vi "Main.vi"() -> ()   [LabVIEW 2022 SP3]
uses:
  <userlib>/_OpenG.lib/file/file.llb/Build Path - File Names Array__ogtk.vi
  <userlib>/_OpenG.lib/file/file.llb/Compare Two Paths - Scalar__ogtk.vi
  <userlib>/_OpenG.lib/file/file.llb/Build Path - Traditional - path__ogtk.vi
  <userlib>/_OpenG.lib/file/file.llb/Strip Path - Traditional__ogtk.vi
panel:
  in  "Status":string
  in  "Abort":bool
  out "Folder Stack":i32
  out "Current File":path
  out "Copied Count":i32
  out "Files Copied":path[](array[path])
  out "error out":errorcluster
  in  "Dest Folder":path=path "\\\\tyrian\\D/Literature/Comics/Marvel"
  in  "Local Folder":path=path "D:/Marvel"
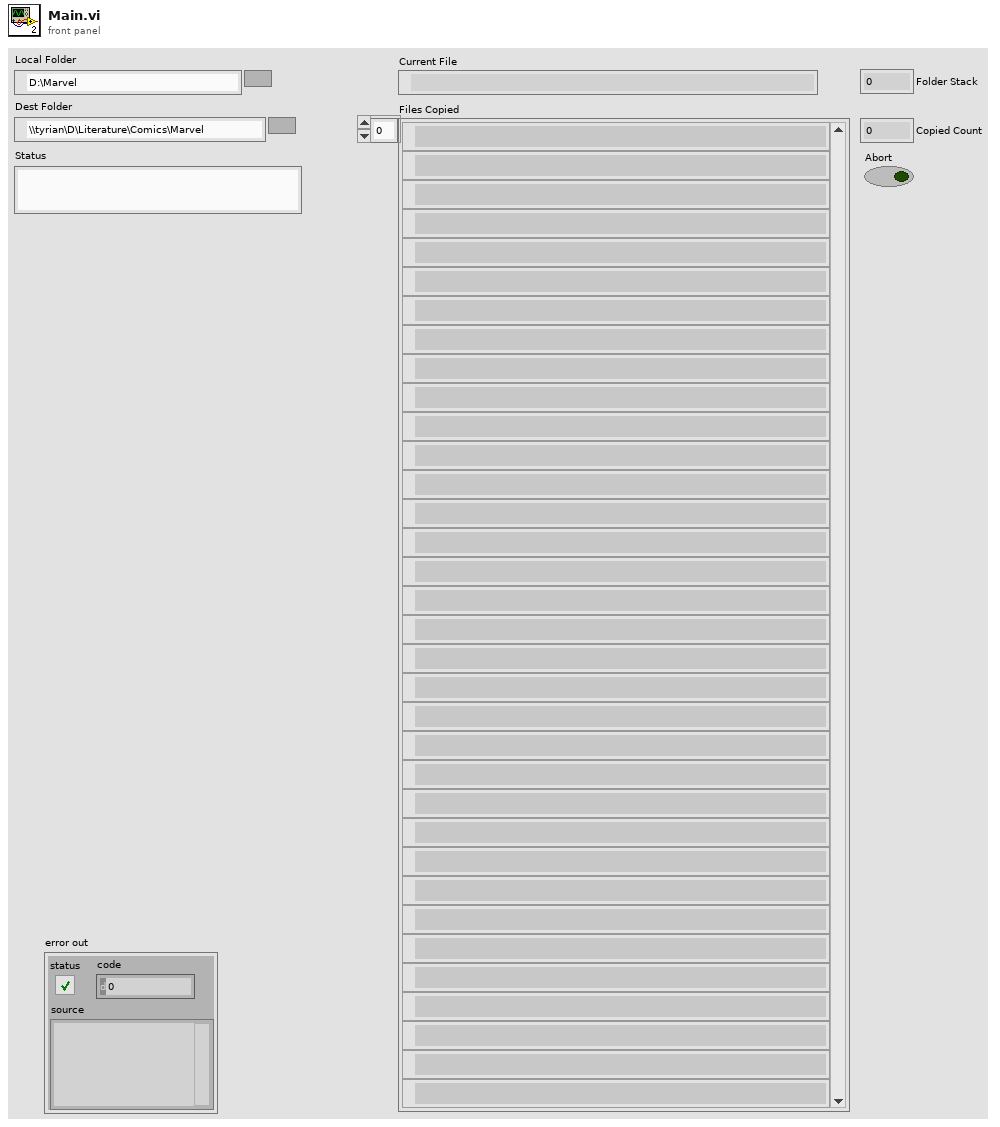
[diagram p1: front panel]
types:
  T1 = cluster{"Archive":bool, "Normal":bool, "Temporary":bool, "Compressed":bool, "Offline":bool, "Content Indexed":bool, "Encrypted (cannot set)":bool}
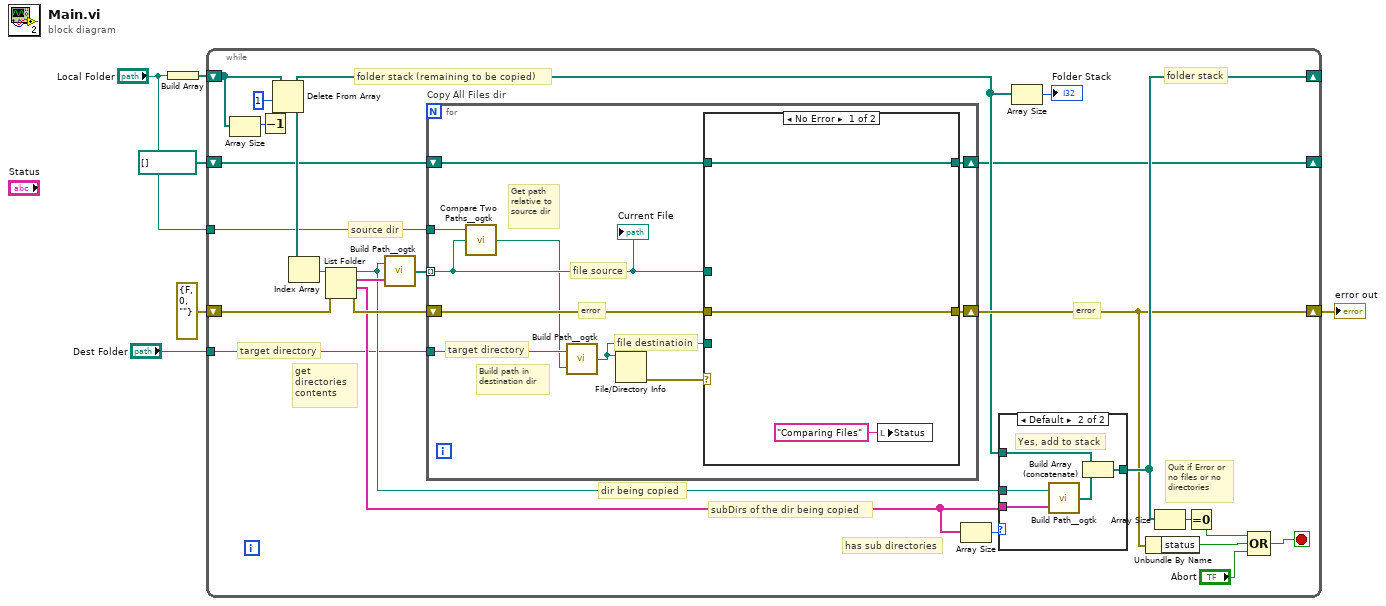
[diagram p0: block diagram]
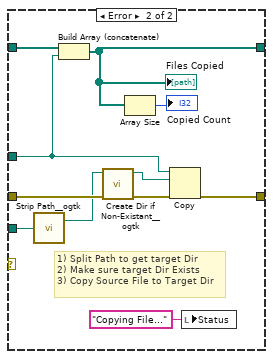
[diagram p3: hidden frame]
diagram:
  n1 = Build Array("Local Folder") -> (w6:path[])
  n2 = while {
    shift-right: [w18] -> _
    shift-left: w6 -> [w21]
    shift-right: [w12] -> w3
    shift-left: errorcluster {"status"=FALSE, "code"=0, "source"=""} ("error out") -> [w22]
    tunnel: "Local Folder" -> [w14]
    tunnel: "Dest Folder" -> [w13]
    shift-right: [w8] -> _
    shift-left: path[] [] -> [w9]
    stop <- w23 stop-if-true
    (unwired) T1 {"Archive"=FALSE, "Normal"=FALSE, "Temporary"=FALSE, "Compressed"=FALSE, "Offline"=FALSE, "Content Indexed"=FALSE, "Encrypted (cannot set)"=FALSE} ("FileAttribute")
    # "folder stack"
    # "error"
    # "target directory"
    # "subDirs of the dir being copied"
    # "dir being copied"
    # "folder stack (remaining to be copied)"
    # "source dir"
    # "get directories contents"
    # "Quit if Error or no files or no directories"
    # "has sub directories"
    n3 = Array Size(array=w21) -> (size(s)=w19:i32)
    n4 = Decrement(x=w19) -> (x-1=w20:i32)
    n5 = Delete From Array(array=w21, length=1 ("Length"), index=w20) -> (deleted portion=w31:path[], array with subset deleted=w11:path[])
    n6 = Index Array(array=w31) -> (element=w30:path)  [unwired: 1 in]
    n7 = List Folder(path=w30, error in=w22) -> (path out=w16:path, filenames=w17:string[], folder names=w27:string[], error out=w29:errorcluster)  [unwired: 2 in]
    n8 = call-poly <userlib>:"Build Path__ogtk.vi"("name or relative path"=w17, "base path"=w16) -> ("appended path"=w15:path[])
    n9 = for "Copy All Files dir" {
      shift-right: [w44] -> w12
      shift-left: w29 -> [w45]
      tunnel: w15 -> [w42] mode=indexing
      tunnel: w14 -> [w43]
      tunnel: w13 -> [w48]
      shift-right: [w39] -> w8
      shift-left: w9 -> [w40]
      # "file destinatioin"
      # "file source"
      # "target directory"
      # "error"
      # "Build path in destination dir"
      # "Get path relative to source dir"
      n10 = call-poly <userlib>:"Compare Two Paths__ogtk.vi"("path2"=w42, "path1"=w43) -> ("relative path from 1 to 2"=w41:path)  [unwired: 1 in, 2 out]
      n11 = call-poly <userlib>:"Build Path__ogtk.vi"("name or relative path"=w41, "base path"=w48) -> ("appended path"=w46:path)
      n12 = File/Directory Info(path=w46) -> (error out=w47:errorcluster)  [unwired: 1 in, 6 out]
      n13 = case "No Error means that file\nalready exists" shown="No Error" w47 {
        tunnel: w46 -> [_ w61]
        tunnel: w42 -> [_ w55]
        tunnel: w45 -> [w51 w60]
        tunnel: [w51 w62] -> w44
        tunnel: w40 -> [w50 w56]
        tunnel: [w50 w53] -> w39
        frame No Error {
          n14 = local write "Status"("Comparing Files" ("Status")) -> ()
        }
        frame Error {
          # "1) Split Path to get target Dir\n2) Make sure target Dir Exists\n3) Copy Source File to Target Dir"
          n15 = call-poly <userlib>:"Strip Path__ogtk.vi"("path"=w61) -> ("stripped path"=w58:path)  [unwired: 1 out]
          n16 = Build Array (concatenate)(w56, w55) -> (w53:path[])
          "Files Copied" <- w53
          n17 = call <userlib>:"Create Dir if Non-Existant__ogtk.vi"("error in (no error)"=w60, "Directory Path"=w58) -> ("error out"=w59:errorcluster, "dup Directory Path"=w57:path)  [unwired: 7 in, 1 out]
          n18 = Array Size(array=w53) -> (size(s)=→"Copied Count":i32)
          n19 = Copy(8:w59, 10:w57, 11:w55) -> (0:w62:errorcluster)  [unwired: 2 in, 2 out]
          n20 = local write "Status"("Copying File..." ("Status")) -> ()
        }
      }
      "Current File" <- w42
    }
    n21 = Array Size(array=w27) -> (size(s)=w28:i32)
    n22 = case shown="Default" w28 {
      tunnel: w16 -> [_ w34]
      tunnel: w27 -> [_ w38]
      tunnel: w11 -> [w33 w36]
      tunnel: [w33 w35] -> w18
      frame 0 {
      }
      frame Default {
        # "Yes, add to stack"
        n23 = call-poly <userlib>:"Build Path__ogtk.vi"("name or relative path"=w38, "base path"=w34) -> ("appended path"=w37:path[])
        n24 = Build Array (concatenate)(w36, w37) -> (w35:path[])
      }
    }
    n25 = Array Size(array=w11) -> (size(s)=→"Folder Stack":i32)
    n26 = Unbundle By Name(w12) -> ("status"=w25:bool)
    n27 = Array Size(array=w18) -> (size(s)=w26:i32)
    n28 = Equal To 0?(x=w26) -> (x = 0?=w24:bool)
    n29 = Compound Arithmetic op=OR(w24, w25, "Abort") -> (w23:bool)
  }
  "error out" <- w3
